vi "Initializer_Valve (SubVI).vi"(11 "VISA Refnum in":refnum<visa-resource-name>) -> ()   [LabVIEW 2020]
uses:
  <vilib>/Instr/_visa.llb/VISA Configure Serial Port (Instr).vi
panel:
  out "read buffer":string
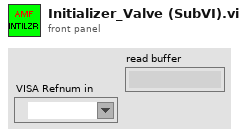
[diagram p1: front panel]
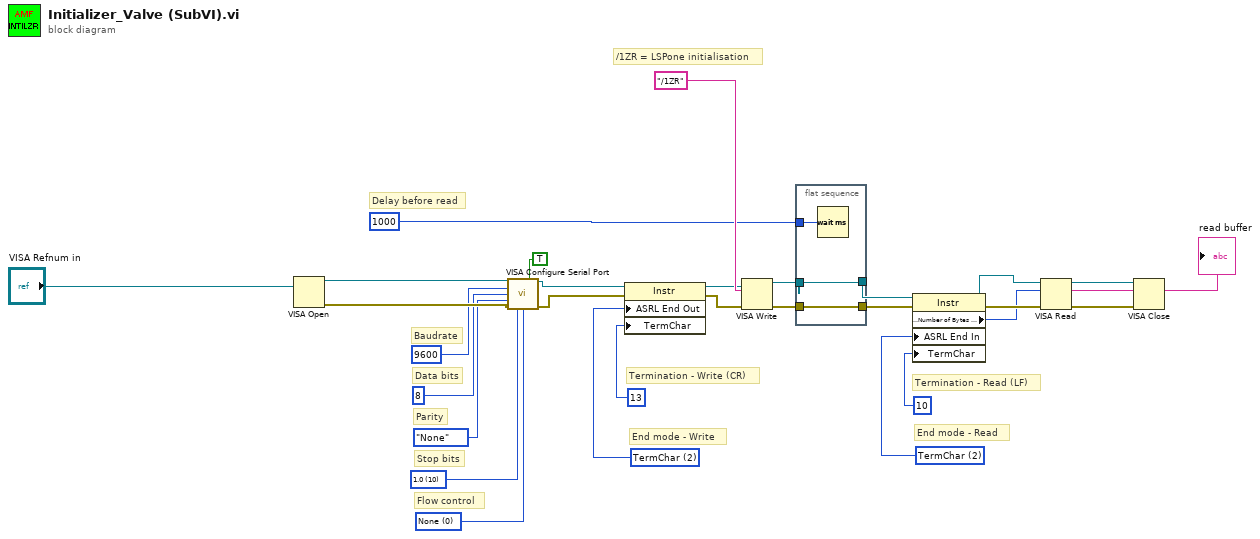
[diagram p0: block diagram]
diagram:
  w2 = u16 2 items=["None", "Last Bit", "TermChar"] ("Serial Settings:End Mode for Reads")
  w5 = u16 2 items=["None", "Last Bit", "TermChar", "Break"] ("Serial Settings:End Mode for Writes")
  w6 = u16 0 items=["None", "XON/XOFF", "RTS/CTS", "XON/XOFF & RTS/CTS", "DTR/DSR", "XON/XOFF & DTR/DSR"] ("flow control (0:none)")
  w7 = u16 10 items=["1.0"=10, "1.5"=15, "2.0"=20] ("stop bits (10: 1 bit)")
  # "/1ZR = LSPone initialisation"
  # "End mode - Read"
  # "Termination - Read (LF)"
  # "End mode - Write"
  # "Termination - Write (CR)"
  # "Flow control"
  # "Stop bits"
  # "Parity"
  # "Data bits"
  # "Baudrate"
  # "Delay before read"
  n1 = VISA Open(VISA resource name="VISA Refnum in") -> (VISA resource name=w15:refnum<visa-resource-name>, error out=w14:errorcluster)  [unwired: 4 in]
  n2 = call-poly "VISA Configure Serial Port"("VISA resource name"=w15, "Enable Termination\nChar (T)"=TRUE, "baud rate (9600)"=u32 9600, "data bits (8)"=u16 8, "parity (0:none)"=enum16{"None", "Odd", "Even", "Mark", "Space"}."None", "error in (no error)"=w14, "stop bits (10: 1 bit)"=w7, "flow control (0:none)"=w6) -> ("VISA resource name out"=w22:refnum<visa-resource-name>, "error out"=w21:errorcluster)  [unwired: 1 in, 5 out]
  n3 = property class="Instr"(reference=w22, error in=w21, "ASRL End Out"=w5, "TermChar"=u8 13 ("Message Based Settings:Termination Character")) -> (reference out=w20:refnum<visa-resource-name>, error out=w19:errorcluster)
  n4 = VISA Write(VISA resource name=w20, write buffer="/1ZR", error in (no error)=w19) -> (VISA resource name out=w26:refnum<visa-resource-name>, error out=w28:errorcluster)  [unwired: 1 out]
  n5 = flat-sequence {
    tunnel: w28 -> [w31]
    tunnel: [w31] -> w27
    tunnel: w26 -> [w30]
    tunnel: [w30] -> w11
    tunnel: u32 1000 ("delay before read (ms)") -> [w32]
    frame #0 {
      n6 = Wait (ms)(milliseconds to wait=w32) -> ()  [unwired: 1 out]
    }
  }
  n7 = property class="Instr"(reference=w11, error in=w27, "ASRL End In"=w2, "TermChar"=u8 10 ("Message Based Settings:Termination Character")) -> (reference out=w12:refnum<visa-resource-name>, error out=w24:errorcluster, "Serial Settings:Number of Bytes at Serial Port"=w23:u32)
  n8 = VISA Read(VISA resource name=w12, byte count=w23, error in (no error)=w24) -> (VISA resource name out=w17:refnum<visa-resource-name>, read buffer=→"read buffer":string, error out=w16:errorcluster)  [unwired: 1 out]
  n9 = VISA Close(VISA resource name=w17, error in (no error)=w16) -> ()  [unwired: 1 out]
